vi "Finish Scan.vi"(8 "error in (no error)":errorcluster, 11 "Magnetic Field Lakeshore Continuous in":refnum<class "Magnetic Field Lakeshore Continuous.lvclass">) -> (0 "error out":errorcluster, 3 "Magnetic Field Lakeshore Continuous out":refnum<class "Magnetic Field Lakeshore Continuous.lvclass">)   [LabVIEW 2017, in "Magnetic Field Lakeshore Continuous.lvclass"]
doc: "(Dynamic) Perform any cleanup after the last step. Restore the instrument to its initial pre-scan state if \"Return to Start\" is true."
uses:
  Magnetic Field Lakeshore Continuous.lvclass
  Scanner/Scanner.lvclass
  Instruments/Utility Classes/Scannable/Scannable.lvclass
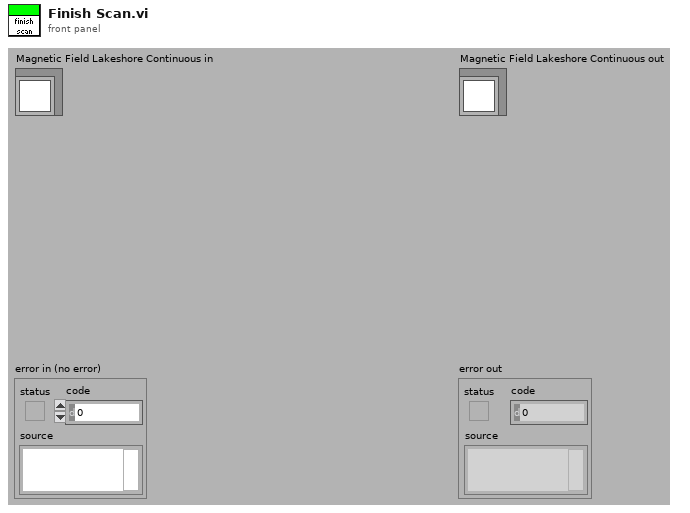
[diagram p1: front panel]
types:
  T1 = typedef "Scanner.lvclass/Range.ctl" = cluster{"xi":dbl, "xf":dbl, "dx":dbl, "Return to...?":bool, "Return to":dbl}
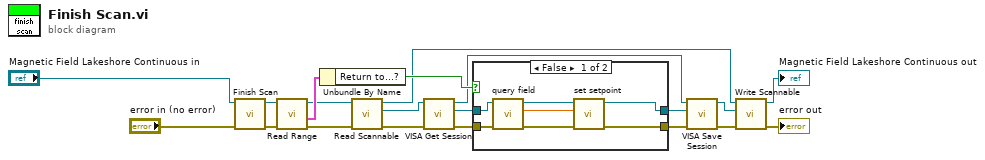
[diagram p0: block diagram]
diagram:
  n1 = call-parent "Finish Scan.vi"("error in (no error)"="error in (no error)", "Scanner in"="Magnetic Field Lakeshore Continuous in") -> ("error out"=w17:errorcluster, "Scanner out"=w18:refnum<class "Magnetic Field Lakeshore Continuous.lvclass">)  [unwired: 8 in]
  n2 = call-dynamic "Read Range.vi"("error in (no error)"=w17, "Scanner.lvclass in"=w18) -> ("error out"=w9:errorcluster, "Range"=w16:T1, "Scanner.lvclass out"=w12:refnum<class "Magnetic Field Lakeshore Continuous.lvclass">)  [unwired: 7 out]
  n3 = Unbundle By Name(w16) -> ("Return to...?"=w15:bool)
  n4 = call-dynamic "Read Scannable.vi"("error in (no error)"=w9, "Scanner.lvclass in"=w12) -> ("error out"=w13:errorcluster, "Scannable.lvclass"=w5:refnum<class "Scannable.lvclass">, "Scanner.lvclass out"=w11:refnum<class "Magnetic Field Lakeshore Continuous.lvclass">)  [unwired: 7 out]
  n5 = call-dynamic "VISA Get Session.vi"("error in (no error)"=w13, "Instrument.lvclass in"=w5) -> ("error out"=w8:errorcluster, "VISA Resource Name"=w2:refnum<visa-resource-name>, "Instrument.lvclass out"=w4:refnum<class "Scannable.lvclass">)  [unwired: 7 out]
  n6 = case shown="False" w15 {
    tunnel: w8 -> [w27 w28]
    tunnel: [w25 w28] -> w7
    tunnel: w2 -> [w24 w29]
    tunnel: [w22 w29] -> w1
    frame False {
      n7 = call "query field.vi"("error in (no error)"=w27, "VISA session"=w24) -> ("error out"=w26:errorcluster, "Field reading"=w21:dbl[unit], "dup VISA session"=w23:refnum<visa-resource-name>)  [unwired: 7 in]
      n8 = call "set setpoint.vi"("error in (no error)"=w26, "Setpoint"=w21, "VISA session"=w23) -> ("error out"=w25:errorcluster, "dup VISA session"=w22:refnum<visa-resource-name>)  [unwired: 7 in]
    }
    frame True {
    }
  }
  n9 = call-dynamic "VISA Save Session.vi"("error in (no error)"=w7, "VISA Resource Name"=w1, "Instrument.lvclass in"=w4) -> ("error out"=w14:errorcluster, "Instrument.lvclass out"=w3:refnum<class "Scannable.lvclass">)  [unwired: 7 out]
  n10 = call-dynamic "Write Scannable.vi"("error in (no error)"=w14, "Scannable.lvclass"=w3, "Scanner.lvclass in"=w11) -> ("error out"=→"error out":errorcluster, "Scanner.lvclass out"=→"Magnetic Field Lakeshore Continuous out":refnum<class "Magnetic Field Lakeshore Continuous.lvclass">)  [unwired: 7 out]
